vi "subbus_mread.vi"(8 "error in (no error)":errorcluster, 9 "Port":string, 11 "Cmd":string) -> (0 "error out":errorcluster, 1 "PortOut":string, 2 "Ack":bool, 3 "Values":u16[](array[numeric]) format="%x")   [LabVIEW 2016]
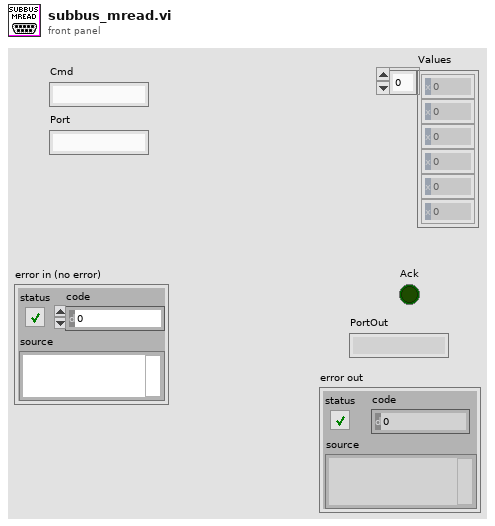
[diagram p1: front panel]
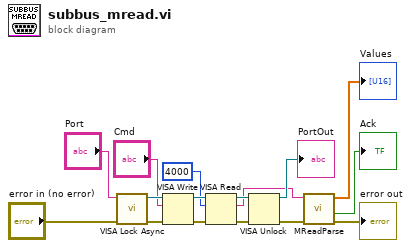
[diagram p0: block diagram]
diagram:
  n1 = call <vilib>:"VISA Lock Async.vi"("error in (no error)"="error in (no error)", "VISA resource name"="Port") -> ("error out"=w13:errorcluster, "VISA resource name out"=w12:refnum<visa-resource-name>)  [unwired: 7 in, 1 out]
  n2 = VISA Write(VISA resource name=w12, write buffer="Cmd", error in (no error)=w13) -> (VISA resource name out=w16:refnum<visa-resource-name>, error out=w15:errorcluster)  [unwired: 1 out]
  n3 = VISA Read(VISA resource name=w16, byte count=4000, error in (no error)=w15) -> (VISA resource name out=w11:refnum<visa-resource-name>, read buffer=w5:string, error out=w10:errorcluster)  [unwired: 1 out]
  n4 = VISA Unlock(8:w10, 11:w11) -> (0:w4:errorcluster, 3:→"PortOut":refnum<visa-resource-name>)
  n5 = call "MReadParse.vi"("error in (no error)"=w4, "StrIn"=w5) -> ("error out"=→"error out":errorcluster, "AllAck"=→"Ack":bool, "Values"=→"Values":dbl[])  [unwired: 6 in, 1 out]
